vi "BMP280.vi"() -> ()   [LabVIEW 2020]
uses:
  <vilib>/MakerHub/LINX/Public/Utilities/Open Local.vi
  Modules/LINX I2C/LINX I2C.lvclass
  Modules/BMP280 PressureSensor/BMP208.lvclass
  <vilib>/MakerHub/LINX/LMH-LINX.lvlib
panel:
  in  "stop":bool
  out "error out":errorcluster
  out "BMP280":cluster{"Temperature":dbl, "Humidity":dbl}(graph)
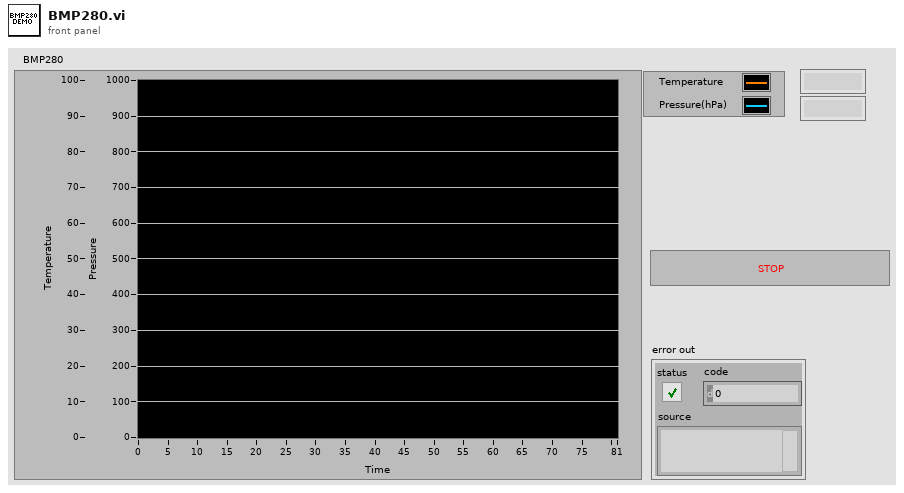
[diagram p1: front panel]
types:
  T1 = typedef "LMH-LINX.lvlib/LINX Ref.ctl" = cluster{"IO":T2, "Interface":T3, "LINX Device Config":T4}
  T2 = typedef "LMH-LINX.lvlib/Platform.ctl" = enum16{"Remote", "Local"}
  T3 = typedef "LMH-LINX.lvlib/Interface.ctl" = enum16{"Serial", "TCP"}
  T4 = typedef "LMH-LINX.lvlib/Device.lvlib/LINX Device Config.ctl" = cluster{"Interface":T3, "COM Port":refnum<visa-resource-name>, "TCP Configuration":T5, "Device Family":u8, "Device ID":u8, "Device Name":string, "TCP Ref":refnum<k5>, "Channels":T6}
  T5 = typedef "LMH-LINX.lvlib/Device.lvlib/TCP Config.ctl" = cluster{"IP Address":string, "Port":u16}
  T6 = typedef "LMH-LINX.lvlib/Channels.ctl" = cluster{"DI":u8[], "DO":u8[], "AI":u8[], "AO":u8[], "PWM":u8[], "QE":u8[], "UART":u8[], "I2C 2":u8[], "SPI":u8[], "CAN":u8[], "Servo":u8[], "AI Ref (V)":dbl, "AI Resolution (Bits)":u8, "AO Ref (V)":dbl, "AO Resolution (Bits)":u8}
  T7 = typedef "BMP208.lvclass/td_cluster_measurements.ctl" = cluster{"Temperature":dbl, "Pressure":dbl}
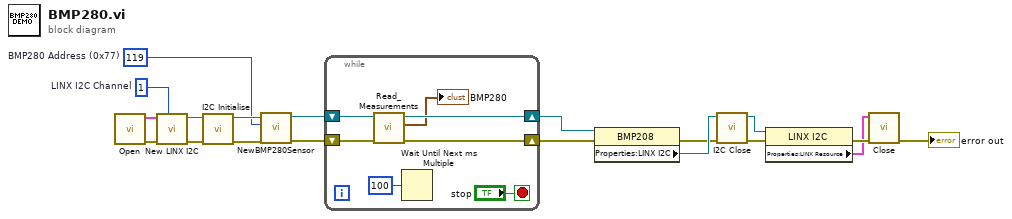
[diagram p0: block diagram]
diagram:
  w1 = u8 1  # LINX I2C Channel
  w9 = u8 119  # BMP280 Address (0x77)
  n1 = call-poly <vilib>:"Open.vi"() -> ("Error Out"=w17:errorcluster, "LINX Resource"=w18:T1)  [unwired: 9 in, 1 out]
  n2 = call "New LINX I2C.vi"("LINX I2C Channel"=w1, "error in (no error)"=w17, "LINX Resource"=w18) -> ("error out"=w15:errorcluster, "LINX I2C out"=w16:refnum<class "LINX I2C.lvclass">)  [unwired: 7 in]
  n3 = call-dynamic "I2C Initialise.vi"("error in (no error)"=w15, "LINX I2C in"=w16) -> ("error out"=w10:errorcluster, "LINX I2C out"=w11:refnum<class "LINX I2C.lvclass">)  [unwired: 8 in]
  n4 = call "NewBMP280Sensor.vi"("error in"=w10, "I2C Slave Addr (0x77)"=w9, "LINX I2C"=w11) -> ("error out"=w8:errorcluster, "BMP208 out"=w4:refnum<class "BMP208.lvclass">)  [unwired: 7 in]
  n5 = while {
    shift-right: [w25] -> w5
    shift-left: w8 -> [w26]
    shift-right: [w23] -> w3
    shift-left: w4 -> [w24]
    stop <- "stop" stop-if-true
    n6 = call "Read_Measurements.vi"("error in (no error)"=w26, "BMP208 in"=w24) -> ("error out"=w25:errorcluster, "Measurements"=→"BMP280":T7, "BMP208 out"=w23:refnum<class "BMP208.lvclass">)  [unwired: 7 in]
    n7 = Wait Until Next ms Multiple(millisecond multiple=u32 100) -> ()  [unwired: 1 out]
  }
  n8 = property class="BMP208"(reference=w3, error in=w5) -> (error out=w6:errorcluster, "Properties:LINX I2C"=w7:refnum<class "LINX I2C.lvclass">)  [unwired: 1 out]
  n9 = call-dynamic "I2C Close.vi"("error in (no error)"=w6, "LINX I2C in"=w7) -> ("error out"=w19:errorcluster, "LINX I2C out"=w13:refnum<class "LINX I2C.lvclass">)  [unwired: 8 in]
  n10 = property class="LINX I2C"(reference=w13, error in=w19) -> (error out=w14:errorcluster, "Properties:LINX Resource"=w2:T1)  [unwired: 1 out]
  n11 = call <vilib>:"Close.vi"("Error In"=w14, "LINX Resource"=w2) -> ("Error Out"=→"error out":errorcluster)  [unwired: 9 in]
